vi "Update Zone.vi"(8 "error in":errorcluster, 9 "Run Selector":bool, 10 "Zone Step":i32, 11 "Zone Setup Array":T2[](array[typedef])) -> (0 "error out":errorcluster, 2 "Zone Step":i32, 3 "Zone Indicators":T1)   [LabVIEW 8.6]
doc: "This VI checks to see whether the specified amount of time has elapsed for the current step. If it has, the timer is reset and the next zone is set. If the \"Run Selector\" is set to Continuous, it will reset to the first step once the end of the array is reached.\n\nThis VI also updates the zone indicators to the correct zone.\n\nNote: No checking is done to see whether the information in the Zone Setup Array is valid. This results in the following behavior:\n- If \"Zone Selector\" is empty or not valid, it will still count through the desired time, but will not show an active zone. This may be considered desired behavior if you wanted to have delays between different steps of the sequence.\n-If \"Timing\" is 0, the current step will be run for 1 iteration, resulting in the corresponding zone indicator to breifly flash. This behavior could be improved by checking for a 0 value and incrementing the step if found, but the author of the VI did not feel this corner case warranted development at this time (due to lack of time for potential debugging). It could always be implemented later."
uses:
  Controls/Timer Actions.ctl
  Controls/Zone Indicators.ctl
  Controls/Zone.ctl
  Controls/Zone Setup.ctl
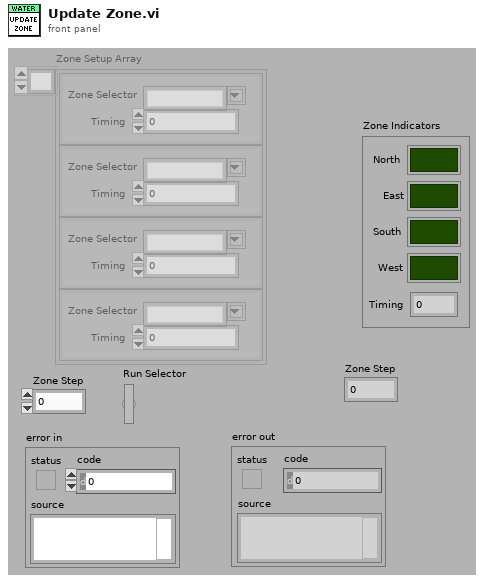
[diagram p1: front panel]
types:
  T1 = typedef "Zone Indicators.ctl" = cluster{"North":bool, "East":bool, "South":bool, "West":bool, "Timing":dbl}
  T2 = typedef "Zone Setup.ctl" = cluster{"Zone Selector":T3, "Timing":u32}
  T3 = typedef "Zone.ctl" = string
  T4 = typedef "Timer Actions.ctl" = enum16{"Reset", "Check Time"}
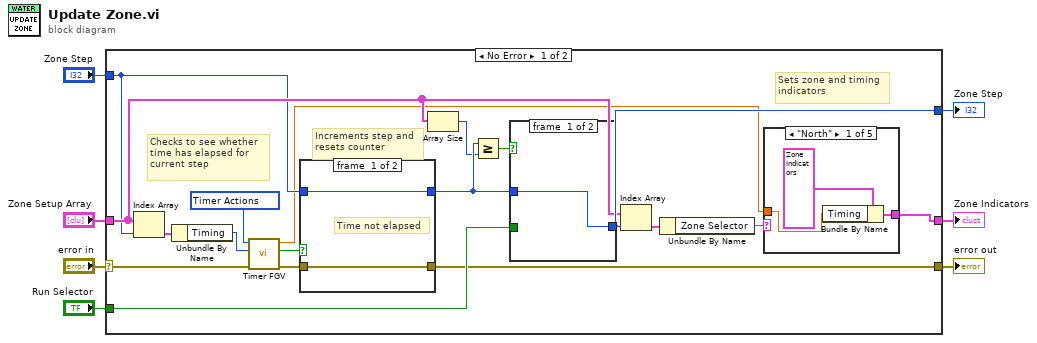
[diagram p0: block diagram]
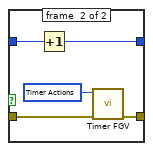
[diagram p2: hidden frame]
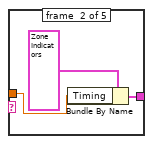
[diagram p3: hidden frame]
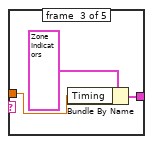
[diagram p4: hidden frame]
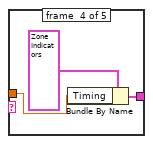
[diagram p5: hidden frame]
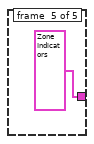
[diagram p6: hidden frame]
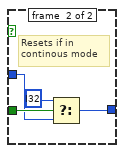
[diagram p7: hidden frame]
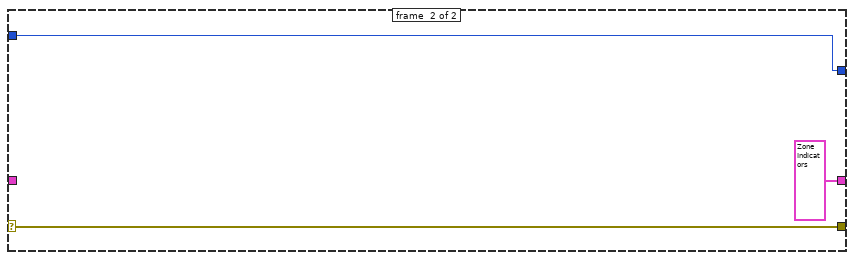
[diagram p8: hidden frame]
diagram:
  n1 = case shown="No Error" "error in" {
    selector: "error in" -> [w22 w53]
    tunnel: [w11 w53] -> w6
    tunnel: "Zone Setup Array" -> [w18 _]
    tunnel: "Zone Step" -> [w12 w52]
    tunnel: [w19 w52] -> w3
    tunnel: "Run Selector" -> [w20 _]
    tunnel: [w15 T1 ? ("Zone Indicators")] -> w1
    frame #0 {
      # "Sets zone and timing\nindicators"
      # "Increments step and\nresets counter"
      # "Checks to see whether\ntime has elapsed for \ncurrent step"
      n2 = Index Array(array=w18, index=w12) -> (element=w24:T2)
      n3 = Unbundle By Name(w24) -> ("Timing"=w25:u32)
      n4 = call "Timer FGV.vi"("error in"=w22, "Timing (s)"=w25, "Timer Action"=T4 ?) -> ("error out"=w14:errorcluster, "Done?"=w13:bool, "Elapsed Time"=w8:dbl)  [unwired: 6 in]
      n5 = case shown="True" w13 {
        tunnel: w14 -> [w26 w32]
        tunnel: w12 -> [w27 w30]
        tunnel: [w27 w29] -> w10
        tunnel: [w26 w28] -> w11
        frame #0 {
          # "Time not elapsed"
        }
        frame #1 {
          n6 = Increment(x=w30) -> (x+1=w29:i32)
          n7 = call "Timer FGV.vi"("error in"=w32, "Timer Action"=T4 ?) -> ("error out"=w28:errorcluster)  [unwired: 7 in, 2 out]
        }
      }
      n8 = Array Size(array=w18) -> (size(s)=w9:i32)
      n9 = Greater Or Equal?(x=w10, y=w9) -> (x >= y?=w21:bool)
      n10 = case shown="True" w21 {
        tunnel: w10 -> [w46 w48]
        tunnel: [w46 w47] -> w19
        tunnel: w20 -> [_ w50]
        frame #0 {
        }
        frame #1 {
          # "Resets if in \ncontinous mode"
          n11 = Select(t=i32 ? ("Zone Step"), s=w50, f=w48) -> (s? t:f=w47:i32)
        }
      }
      n12 = Index Array(array=w18, index=w19) -> (element=w17:T2)
      n13 = Unbundle By Name(w17) -> ("Zone Selector"=w16:T3)
      n14 = case shown="\"North\"" w16 {
        tunnel: [w34 w37 w40 w43 T1 ? ("Zone Indicators")] -> w15
        tunnel: w8 -> [w33 w36 w39 w42 _]
        frame #0 {
          n15 = Bundle By Name(cluster=T1 ? ("Zone Indicators"), "Timing"=w33) -> (w34:T1)
        }
        frame #1 {
          n16 = Bundle By Name(cluster=T1 ? ("Zone Indicators"), "Timing"=w36) -> (w37:T1)
        }
        frame #2 {
          n17 = Bundle By Name(cluster=T1 ? ("Zone Indicators"), "Timing"=w39) -> (w40:T1)
        }
        frame #3 {
          n18 = Bundle By Name(cluster=T1 ? ("Zone Indicators"), "Timing"=w42) -> (w43:T1)
        }
        frame #4 {
        }
      }
    }
    frame #1 {
    }
  }
  "error out" <- w6
  "Zone Indicators" <- w1
  "Zone Step" <- w3
